vi "Configure Sweep (Spectrum Monitor).vi"(0 "VISA resource name":refnum<visa-resource-name>, 1 "Stop/Span (1.0075E9 Hz)":dbl=1007500000.0 format="%^#_9g", 7 "Sweep Type (1: Center/Span)":enum16{"Start/Stop", "Center/Span"}(ring)=enum."Center/Span", 9 "Start/Center (3E9 Hz)":dbl=3000000000.0 format="%^#_9g", 11 "error in (no error)":errorcluster) -> (4 "VISA resource name out":refnum<visa-resource-name>, 15 "error out":errorcluster)   [LabVIEW 2011, in "Agilent E5052X.lvlib"]
doc: "Sets the range in which measurements will be taken for the Spectrum measurement.\n\n<b>Note:</b>\n\n1) \"Configure Measurement Characteristics(Spectrum)\" VI must be run before this VI."
uses:
  Agilent E5052X.lvlib
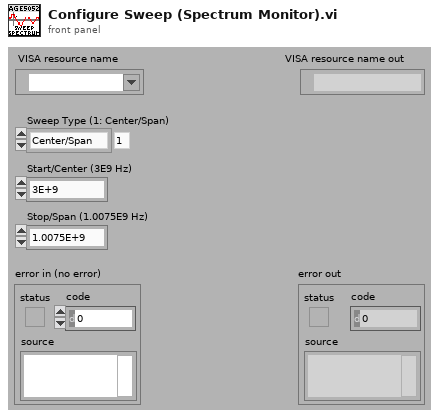
[diagram p1: front panel]
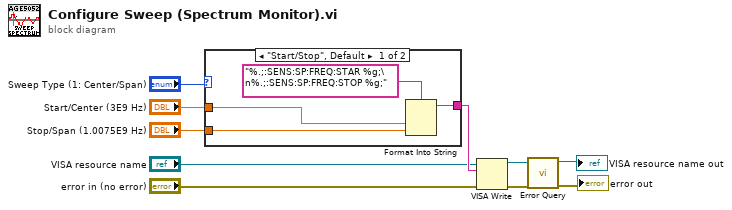
[diagram p0: block diagram]
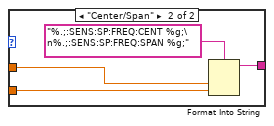
[diagram p2: hidden frame]
diagram:
  n1 = case shown="\"Start/Stop\", Default" "Sweep Type (1: Center/Span)" {
    tunnel: "Start/Center (3E9 Hz)" -> [w13 w17]
    tunnel: "Stop/Span (1.0075E9 Hz)" -> [w14 w16]
    tunnel: [w11 w15] -> w7
    frame "Start/Stop", Default {
      n2 = Format Into String(format string="%.;:SENS:SP:FREQ:STAR %g;\n%.;:SENS:SP:FREQ:STOP %g;", w13, w14) -> (resulting string=w11:string)  [unwired: 2 in, 1 out]
    }
    frame "Center/Span" {
      n3 = Format Into String(format string="%.;:SENS:SP:FREQ:CENT %g;\n%.;:SENS:SP:FREQ:SPAN %g;", w17, w16) -> (resulting string=w15:string)  [unwired: 2 in, 1 out]
    }
  }
  n4 = VISA Write(VISA resource name="VISA resource name", write buffer=w7, error in (no error)="error in (no error)") -> (VISA resource name out=w6:refnum<visa-resource-name>, error out=w5:errorcluster)  [unwired: 1 out]
  n5 = call "Error Query.vi"("error in (no error)"=w5, "VISA resource name"=w6) -> ("error out"=→"error out":errorcluster, "VISA resource name out"=→"VISA resource name out":refnum<visa-resource-name>)  [unwired: 6 in, 2 out]
